vi "SD Write Numeric Array.vi"(8 "error in":errorcluster, 9 "Numeric Array":dbl[](array[numeric]), 10 "Table Prefix":string="SmartDashboard", 11 "Name":string="Numeric Array") -> (0 "error out":errorcluster, 2 "Table Prefix out":string)   [LabVIEW 2017]
doc: "Write the double precision numeric data to the SmartDashboard entry -- /prefix/name."
uses:
  <vilib>/Rock Robotics/Network Tables/Field Data.ctl
  <vilib>/Rock Robotics/Network Tables/Field Type.ctl
  <vilib>/Rock Robotics/Network Tables/Sequence.ctl
  <vilib>/Rock Robotics/Network Tables/Write Value Core.vi
  <vilib>/Rock Robotics/Network Tables/Manage Dirty Field ID List.vi
  <vilib>/Rock Robotics/Network Tables/NT Globals.vi
  <vilib>/Rock Robotics/Network Tables/Update Other Clients.vi
  <vilib>/Rock Robotics/Network Tables/Build Entry Assign Buffer.vi
  <vilib>/Rock Robotics/Network Tables/Field Data Manager.vi
  <vilib>/Rock Robotics/Network Tables/Usage Statistics.vi
  <vilib>/Rock Robotics/Network Tables/Table Manager.vi
  <vilib>/Rock Robotics/Network Tables/Prepare Table Name.vi
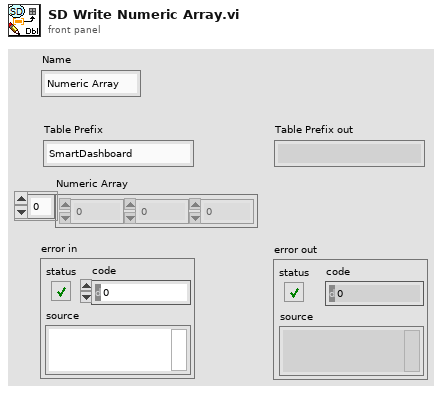
[diagram p1: front panel]
types:
  T1 = typedef "Field Data.ctl" = cluster{"Dbl":dbl, "String":string, "Type":T2, "Boolean":bool, "Sequence #":T3, "Flags":u8}
  T2 = typedef "Field Type.ctl" = enum8{"Invalid", "Bool", "Numeric", "String", "Raw", "Boolean Array", "Numeric Array", "String Array", "RPC"}
  T3 = typedef "Sequence.ctl" = u16
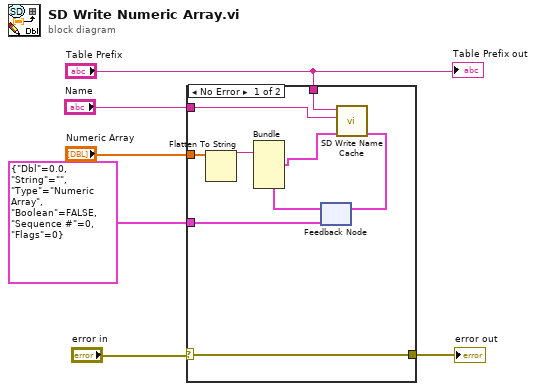
[diagram p0: block diagram]
diagram:
  n1 = case shown="No Error" "error in" {
    selector: "error in" -> [w7 w16]
    tunnel: T1 {"Dbl"=0.0, "String"="", "Type"=enum."Numeric Array", "Boolean"=FALSE, "Sequence #"=0, "Flags"=0} ("Field Value In") -> [w13 _]
    tunnel: "Table Prefix" -> [w11 _]
    tunnel: "Name" -> [w10 _]
    tunnel: "Numeric Array" -> [w8 _]
    tunnel: [w7 w16] -> w1
    frame No Error {
      n2 = Flatten To String(anything=w8) -> (data string=w9:string)  [unwired: 3 in, 2 out]
      n3 = feedback #1(w13) -> (w12:T1)
      n4 = Bundle(cluster=w12, "String"=w9) -> (w14:T1)  [unwired: 5 in]
      n5 = call <vilib>:"SD Write Name Cache.vi"("Field Value In"=w14, "Name"=w10, "Table Prefix"=w11) -> ("Field Value Out"=w15:T1)  [unwired: 8 in]
      n6 = feedback-in #1(w15) -> ()
    }
    frame Error {
    }
  }
  "error out" <- w1
  "Table Prefix out" <- "Table Prefix"
